vi "GenerateAxes.vi"(0 "Text In":string, 2 "Frame":T1={"nx"=1.0, "ny"=0.0, "nz"=0.0, "nw"=0.0, "ox"=0.0, "oy"=1.0, "oz"=0.0, "ow"=0.0, "ax"=0.0, "ay"=0.0, "az"=1.0, "aw"=0.0, "Px"=0.0, "Py"=0.0, "Pz"=0.0, "Pw"=1.0} {"Pw" format="%.2f"; "Pz" format="%.2f"; "Py" format="%.2f"; "Px" format="%.2f"; "aw" format="%.2f"; "az" format="%.2f"; "ay" format="%.2f"; "ax" format="%.2f"; "ow" format="%.2f"; "nw" format="%.2f"; "oz" format="%.2f"; "oy" format="%.2f"; "ox" format="%.2f"; "nz" format="%.2f"; "ny" format="%.2f"; "nx" format="%.2f"}, 3 "Colors":T2={"X Color"=16716800, "Y Color"=1233407, "Z Color"=1441536}, 4 "Show Axis Labels?":bool=TRUE) -> (5 "Text Out":string="Transform {\nchildren [\nShape {\nappearance Appearance {\nmaterial Material {\nemissiveColor 1.00 0.08 0.00\n}\n}\ngeometry IndexedLineSet {\ncoord Coordinate {\npoint [\n0.00 0.00 0.00,1.00 0.00 0.00]}\ncoordIndex [0, 1\r]}},\nShape {\nappearance Appearance {\nmaterial Material {\nemissiveColor 0.07 0.82 1.00\n}\n}\ngeometry IndexedLineSet {\ncoord Coordinate {\npoint [\n0.00 0.00 0.00,0.00 1.00 0.00]}\ncoordIndex [0, 1\r]}},\nShape {\nappearance Appearance {\nmaterial Material {\nemissiveColor 0.08 1.00 0.00\n}\n}\ngeometry IndexedLineSet {\ncoord Coordinate {\npoint [\n0.00 0.00 0.00,0.00 0.00 1.00]}\ncoordIndex [0, 1\r]}}\r\n]}Transform {\ntranslation 1.10 0.00 0.00\nchildren [\nShape {\nappearance Appearance {\nmaterial Material {\nemissiveColor 1.00 0.08 0.00\n}\n}\ngeometry IndexedLineSet {\ncoord Coordinate {\npoint [\n-0.05 0.05 0.00,0.05 -0.05 0.00,0.00 0.00 0.00,0.05 0.05 0.00,-0.05 -0.05 0.00]}\ncoordIndex [0, 1, 2, 3, 4\r]}}\r\n]}Transform {\ntranslation 0.00 1.10 0.00\nchildren [\nShape {\nappearance Appearance {\nmaterial Material {\nemissiveColor 0.07 0.82 1.00\n}\n}\ngeometry IndexedLineSet {\ncoord Coordinate {\npoint [\n-0.05 0.05 0.00,0.00 0.00 0.00,0.05 0.05 0.00,0.00 0.00 0.00,0.00 -0.05 0.00]}\ncoordIndex [0, 1, 2, 3, 4\r]}}\r\n]}Transform {\ntranslation 0.00 0.00 1.10\nchildren [\nShape {\nappearance Appearance {\nmaterial Material {\nemissiveColor 0.08 1.00 0.00\n}\n}\ngeometry IndexedLineSet {\ncoord Coordinate {\npoint [\n-0.05 0.05 0.00,0.05 0.05 0.00,-0.05 -0.05 0.00,0.05 -0.05 0.00]}\ncoordIndex [0, 1, 2, 3\r]}}\r\n]}")   [LabVIEW 2010]
uses:
  ReferenceFrame.ctl
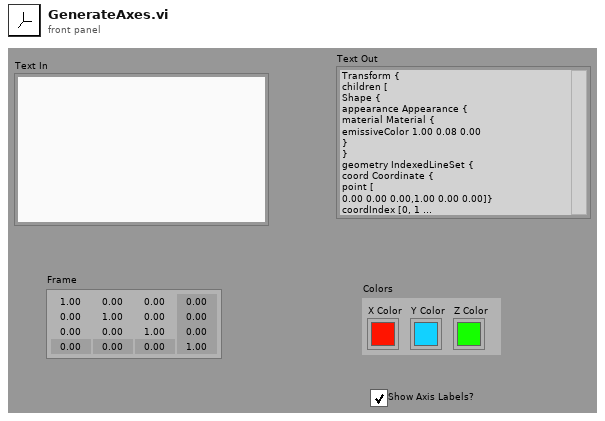
[diagram p1: front panel]
types:
  T1 = typedef "ReferenceFrame.ctl" = cluster{"nx":dbl, "ny":dbl, "nz":dbl, "nw":dbl, "ox":dbl, "oy":dbl, "oz":dbl, "ow":dbl, "ax":dbl, "ay":dbl, "az":dbl, "aw":dbl, "Px":dbl, "Py":dbl, "Pz":dbl, "Pw":dbl}
  T2 = cluster{"X Color":u32, "Y Color":u32, "Z Color":u32}
  T3 = cluster{"X":sgl, "Y":sgl, "Z":sgl, "roll":sgl, "pitch":sgl, "yaw":sgl}
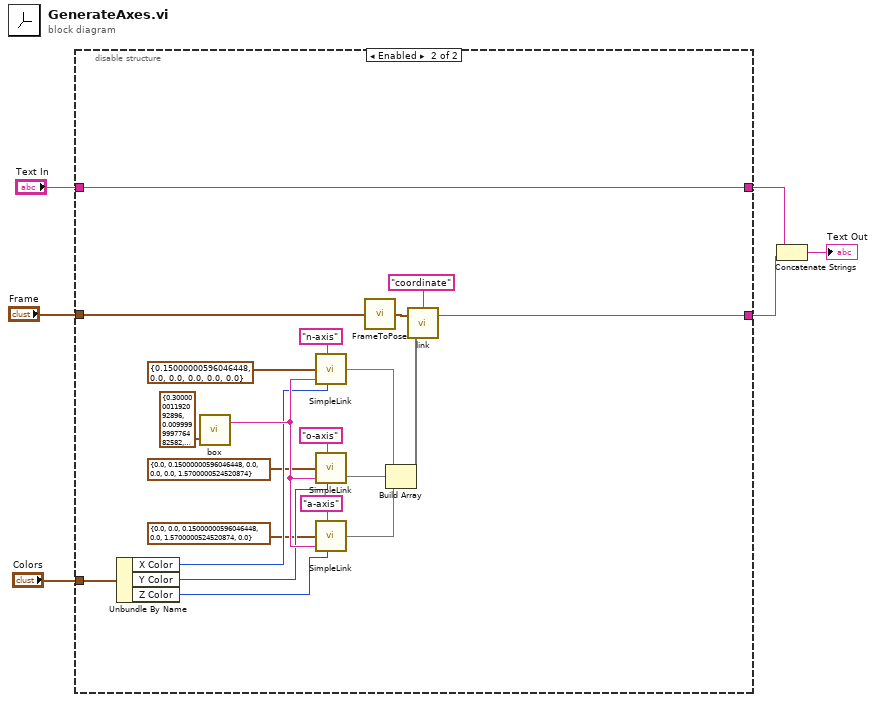
[diagram p0: block diagram]
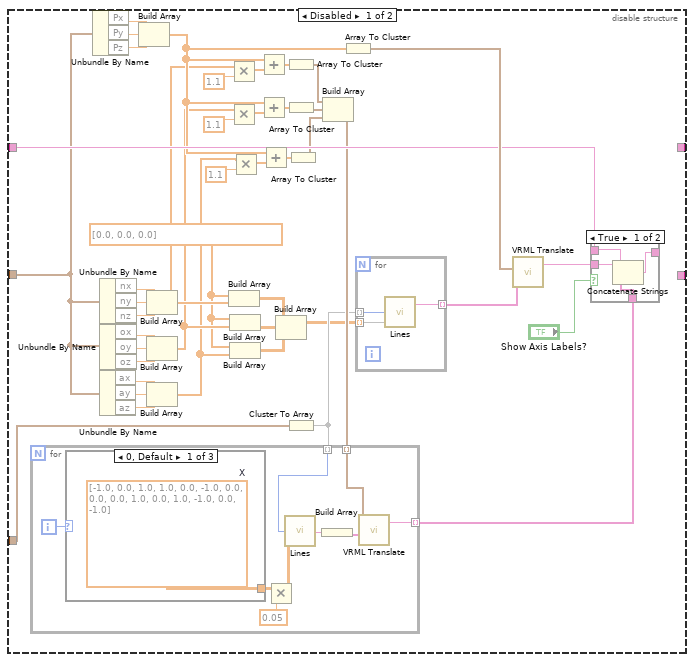
[diagram p2: hidden frame]
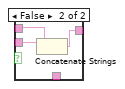
[diagram p3: hidden frame]
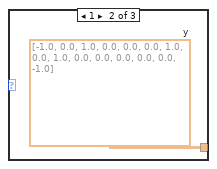
[diagram p4: hidden frame]
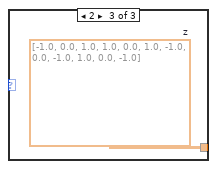
[diagram p5: hidden frame]
diagram:
  n1 = disable-structure shown="Enabled" {
    disable-tunnel: "Text In" -> [w47 w72]
    disable-tunnel: "Frame" -> [w23 w73]
    disable-tunnel: "Colors" -> [w18 w87]
    disable-tunnel: [_ w81] -> w2
    disable-tunnel: [_ w72] -> w3
    frame Disabled {
      w15 = dbl[] [0.0, 0.0, 0.0] ("Data In (XYZ)")
      n2 = Unbundle By Name(w23) -> ("Px"=w41:dbl, "Py"=w42:dbl, "Pz"=w43:dbl)
      n3 = Unbundle By Name(w23) -> ("nx"=w46:dbl, "ny"=w45:dbl, "nz"=w44:dbl)
      n4 = Unbundle By Name(w23) -> ("ox"=w27:dbl, "oy"=w28:dbl, "oz"=w29:dbl)
      n5 = Unbundle By Name(w23) -> ("ax"=w26:dbl, "ay"=w25:dbl, "az"=w24:dbl)
      n6 = Build Array(w41, w42, w43) -> (w40:dbl[])
      n7 = Build Array(w46, w45, w44) -> (w17:dbl[])
      n8 = Build Array(w27, w28, w29) -> (w16:dbl[])
      n9 = Build Array(w26, w25, w24) -> (w14:dbl[])
      n10 = Multiply(x=w17, y=1.1 ("Numeric")) -> (x*y=w36:dbl[])
      n11 = Multiply(x=w16, y=1.1 ("Numeric")) -> (x*y=w35:dbl[])
      n12 = Build Array(w15, w17) -> (w13:dbl[][])
      n13 = Build Array(w15, w16) -> (w12:dbl[][])
      n14 = Build Array(w15, w14) -> (w11:dbl[][])
      n15 = Multiply(x=w14, y=1.1 ("Numeric")) -> (x*y=w30:dbl[])
      n16 = Add(x=w40, y=w36) -> (x+y=w39:dbl[])
      n17 = Add(x=w40, y=w35) -> (x+y=w33:dbl[])
      n18 = Add(x=w40, y=w30) -> (x+y=w32:dbl[])
      n19 = Build Array(w13, w12, w11) -> (w9:dbl[][][])
      n20 = Array To Cluster(array=w39) -> (cluster=w22:cluster{"[0]":dbl, "[1]":dbl, "[2]":dbl})
      n21 = Array To Cluster(array=w33) -> (cluster=w21:cluster{"[0]":dbl, "[1]":dbl, "[2]":dbl})
      n22 = Cluster To Array(cluster=w18) -> (array=w10:u32[])
      n23 = Array To Cluster(array=w32) -> (cluster=w20:cluster{"[0]":dbl, "[1]":dbl, "[2]":dbl})
      n24 = Build Array(w22, w21, w20) -> (w19:cluster{"[0]":dbl, "[1]":dbl, "[2]":dbl}[])
      n25 = for {
        tunnel: [w66] -> w38 mode=indexing
        tunnel: w19 -> [w62] mode=indexing
        tunnel: w10 -> [w60] mode=indexing
        i -> [w61]
        n26 = case shown="0, Default" w61 {
          tunnel: [w69 w70 w71] -> w64
          frame 0, Default {
            w69 = dbl[][] [[-1.0, 0.0, 1.0], [1.0, 0.0, -1.0], [0.0, 0.0, 0.0], [1.0, 0.0, 1.0], [-1.0, 0.0, -1.0]]  # X
          }
          frame 1 {
            w70 = dbl[][] [[-1.0, 0.0, 1.0], [0.0, 0.0, 0.0], [1.0, 0.0, 1.0], [0.0, 0.0, 0.0], [0.0, 0.0, -1.0]]  # y
          }
          frame 2 {
            w71 = dbl[][] [[-1.0, 0.0, 1.0], [1.0, 0.0, 1.0], [-1.0, 0.0, -1.0], [1.0, 0.0, -1.0]]  # z
          }
        }
        n27 = Multiply(x=w64, y=0.05 ("Numeric")) -> (x*y=w63:dbl[][])
        n28 = call "Lines.vi"("emissiveColor"=w60, "Data In (XYZ)"=w63) -> ("Text"=w68:string)  [unwired: 3 in, 1 out]
        n29 = Build Array(w68) -> (w67:string[])
        n30 = call "VRML Translate.vi"("Translation"=w62, "Children"=w67) -> ("Text"=w66:string)  [unwired: 3 in, 1 out]
      }
      n31 = Array To Cluster(array=w40) -> (cluster=w49:cluster{"[0]":dbl, "[1]":dbl, "[2]":dbl})
      n32 = for {
        tunnel: w10 -> [w59] mode=indexing
        tunnel: w9 -> [w58] mode=indexing
        tunnel: [w57] -> w8 mode=indexing
        n33 = call "Lines.vi"("emissiveColor"=w59, "Data In (XYZ)"=w58) -> ("Text"=w57:string)  [unwired: 3 in, 1 out]
      }
      n34 = call "VRML Translate.vi"("Translation"=w49, "Children"=w8) -> ("Text"=w48:string)  [unwired: 3 in, 1 out]
      n35 = case shown="True" "Show Axis Labels?" {
        tunnel: w48 -> [w53 w56]
        tunnel: w47 -> [w52 w55]
        tunnel: [w51 w54] -> _
        tunnel: w38 -> [w50 _]
        frame True {
          n36 = Concatenate Strings(w52, w53, w50) -> (w51:string)
        }
        frame False {
          n37 = Concatenate Strings(w55, w56) -> (w54:string)
        }
      }
    }
    frame Enabled {
      n38 = Unbundle By Name(w87) -> ("X Color"=w86:u32, "Y Color"=w85:u32, "Z Color"=w84:u32)
      n39 = call "box.vi"("Box"=cluster{"Length":sgl, "Width":sgl, "Height":sgl} {"Length"=0.3, "Width"=0.01, "Height"=0.01}) -> ("urdf out"=w88:string)  [unwired: 3 in]
      n40 = call "SimpleLink.vi"("Name"="n-axis", "origin"=T3 {"X"=0.15, "Y"=0.0, "Z"=0.0, "roll"=0.0, "pitch"=0.0, "yaw"=0.0} ("Pose"), "mass"=w88, "link color"=w86) -> (6:w80)  [unwired: 1 in, 1 out]
      n41 = call "SimpleLink.vi"("Name"="o-axis", "origin"=T3 {"X"=0.0, "Y"=0.15, "Z"=0.0, "roll"=0.0, "pitch"=0.0, "yaw"=1.57} ("Pose"), "mass"=w88, "link color"=w85) -> (6:w79)  [unwired: 1 in, 1 out]
      n42 = call "SimpleLink.vi"("Name"="a-axis", "origin"=T3 {"X"=0.0, "Y"=0.0, "Z"=0.15, "roll"=0.0, "pitch"=1.57, "yaw"=0.0} ("Pose"), "mass"=w88, "link color"=w84) -> (6:w78)  [unwired: 1 in, 1 out]
      n43 = call "FrameToPose.vi"("Frame"=w73) -> ("Pose"=w77:T3)
      n44 = Build Array(w80, w79, w78) -> (w83:void[])
      n45 = call "link.vi"("Attributes"=w83, 2:w77, "Name"="coordinate") -> ("urdf out"=w81:string)  [unwired: 1 in]
    }
  }
  n46 = Concatenate Strings(w3, w2) -> (→"Text Out":string)
